vi "Pockels Cal-Message window.vi"(7 "Colour":u32(colorbox)=16777225, 8 "error in (no error)":errorcluster, 10 "Objective index":i32) -> (0 "error out":errorcluster, 1 "Cancelled (Left button pressed)":bool, 3 "Finish":bool)   [LabVIEW 2013]
doc: "Use this template to create a dialog box with event handling."
uses:
  <vilib>/Utility/miscctls.llb/LVPointTypeDef.ctl
  Global Variables/General Globals.vi
panel:
  in  "Finish":bool
  in  "Left Button":bool
  in  "Rigth Button":bool
  out "Message":string="OPTIONAL STEP\nCreate pockels calibration curve for the \n\"Olympus 20X\" objective?\n\nThis curve will be added to the pockels calibration file for information purposes only. It will not be used by the software for anything other than calculating the power shown in the indicator next to the laser power setting knob.\n\nSelect \"No, Finish\" if you don't want to create any additional calibration curves for any of the available objectives.\n\nSelect \"Skip this objective\" if you would like to create calibration curves for one or more of the available objectives other than the one mentioned above.\n\nSelect \"Yes, Calibrate\" if you want to create a calibration curve for the objective mentioned above.\n"
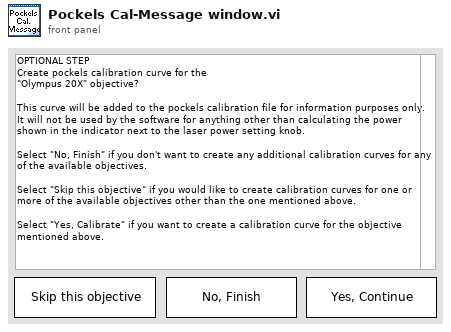
[diagram p1: front panel]
types:
  T1 = typedef "LVPointTypeDef.ctl" = cluster{"Horizontal":i16, "Vertical":i16}
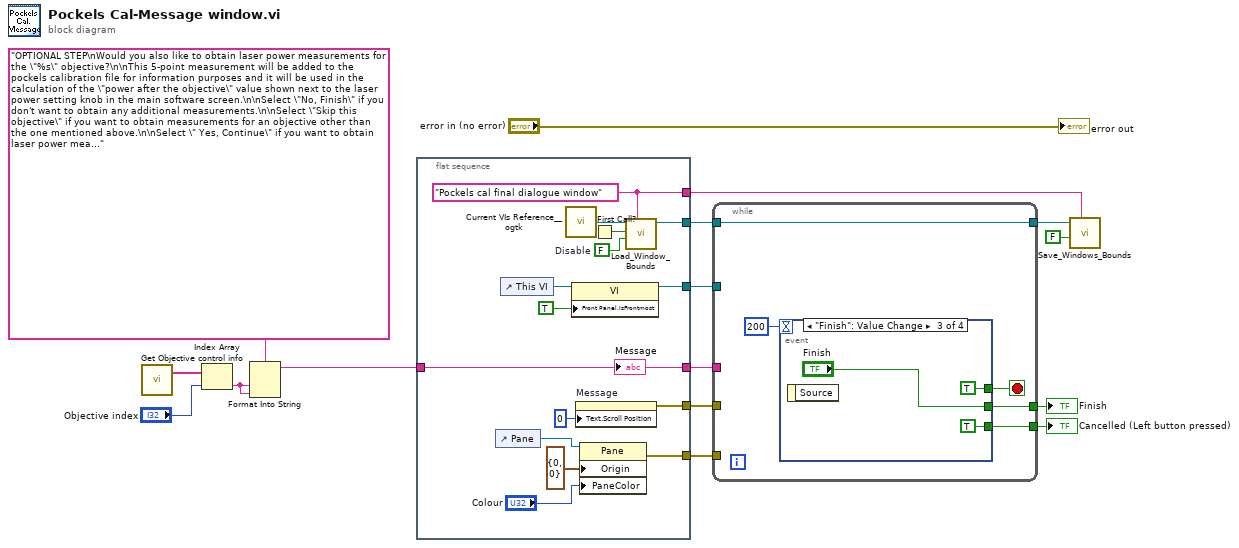
[diagram p0: block diagram]
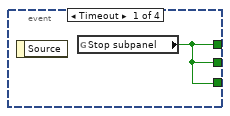
[diagram p2: hidden frame]
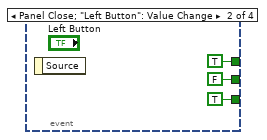
[diagram p3: hidden frame]
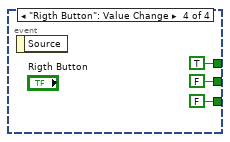
[diagram p4: hidden frame]
diagram:
  n1 = call "Get Objective control info.vi"() -> ("Objective values/strings"=w2:string[])  [unwired: 7 in, 4 out]
  n2 = Index Array(array=w2, index="Objective index") -> (element=w1:string)
  n3 = Format Into String(format string="OPTIONAL STEP\nWould you also like to obtain laser power measurements for the \"%s\" objective?\n\nThis 5-point measurement will be added to the pockels calibration file for information purposes and it will be used in the calculation of the \"power after the objective\" value shown next to the laser power setting knob in the main software screen.\n\nSelect \"No, Finish\" if you don't want to obtain any additional measurements.\n\nSelect \"Skip this objective\" if you want to obtain measurements for an objective other than the one mentioned above.\n\nSelect \" Yes, Continue\" if you want to obtain laser power measurements with the \"%s\" objective fitted.\n", w1, w1) -> (resulting string=w4:string)  [unwired: 2 in, 1 out]
  n4 = flat-sequence {
    tunnel: [w17] -> w16
    tunnel: [w30] -> w15
    tunnel: [w27] -> w14
    tunnel: [w25] -> w13
    tunnel: [w20] -> w11
    tunnel: [w19] -> w9
    tunnel: w4 -> [w17]
    frame #0 {
      w21 = FALSE  # Disable
      w20 = "Pockels cal final dialogue window" ("Window Name (i.e. Key)")
      n5 = control-ref of="Pane"() -> (w24:refnum<vi>)
      n6 = control-ref of="This VI"() -> (w28:refnum<vi>)
      n7 = call "Current VIs Reference__ogtk.vi"() -> ("Current VI's reference"=w23:refnum<vi>)  [unwired: 5 in]
      n8 = property on="Property Node" class="VI"(reference=w28, "Front Panel.IsFrontmost"=TRUE ("Front Panel Window:Is Frontmost")) -> (reference out=w27:refnum<vi>)  [unwired: 1 in, 1 out]
      n9 = property on="Message" class="Str"("Text.Scroll Position"=u32 0) -> (error out=w30:errorcluster)  [unwired: 2 in, 1 out]
      n10 = property class="Pane"(reference=w24, "Origin"=T1 {"Horizontal"=0, "Vertical"=0}, "PaneColor"="Colour") -> (error out=w25:errorcluster)  [unwired: 1 in, 1 out]
      n11 = First Call?() -> (First Call?: T/F=w22:bool)
      n12 = call "Load_Window_Bounds.vi"("Window Name (i.e. Key)"=w20, "Disable"=w21, "First Call"=w22, "Window VI's Ref"=w23) -> ("reference out"=w19:refnum<vi>)  [unwired: 4 in, 3 out]
      "Message" <- w17
    }
  }
  n13 = while {
    tunnel: w16 -> [_]
    tunnel: w15 -> [_]
    tunnel: w13 -> [_]
    tunnel: w14 -> [_]
    tunnel: [w34] -> w12
    tunnel: w9 -> [w33]
    tunnel: [w33] -> w8
    tunnel: [w32] -> w6
    stop <- w36 stop-if-true
    n14 = event shown="[2] \"Finish\": Value Change" {
      selector: _ -> [_ _ _ _]
      dyn-events: _ -> [_ _ _ _]
      timeout: 200 -> [_ _ _ _]
      tunnel: [w37 TRUE ("Stop?") TRUE ("Stop?") TRUE ("Stop?")] -> w36
      tunnel: [w37 TRUE ("Stop subpanel") TRUE ("Stop subpanel") FALSE ("Stop subpanel")] -> w34
      tunnel: [w37 FALSE ("Finish") "Finish" FALSE ("Finish")] -> w32
      event Timeout {
        n15 = event-data() -> ()  [unwired: 1 in, 1 out]
        n16 = global read "General Globals.vi" "Stop subpanel"() -> (w37:bool)
      }
      event Panel Close; "Left Button": Value Change {
        n17 = event-data() -> ()  [unwired: 1 in, 1 out]
      }
      event "Finish": Value Change {
        n18 = event-data() -> ()  [unwired: 1 in, 1 out]
      }
      event "Rigth Button": Value Change {
        n19 = event-data() -> ()  [unwired: 1 in, 1 out]
      }
    }
  }
  "Cancelled (Left button pressed)" <- w12
  "Finish" <- w6
  n20 = call "Save_Windows_Bounds.vi"("Window Name (i.e. Key)"=w11, "Front Panel Window:Open"=FALSE, "Window VI's Ref"=w8) -> ()  [unwired: 8 in, 1 out]
  "error out" <- "error in (no error)"
